vi "Destructor.vi"(8 "error in (no error)":errorcluster, 11 "Mouse in":refnum<class "Mouse.lvclass">) -> (0 "error out":errorcluster)   [LabVIEW 2021, in "InputDevice.lvlib" / "Mouse.lvclass"]
uses:
  Mouse.lvclass
  <vilib>/Utility/inputDevices.llb/closeMouse.vi
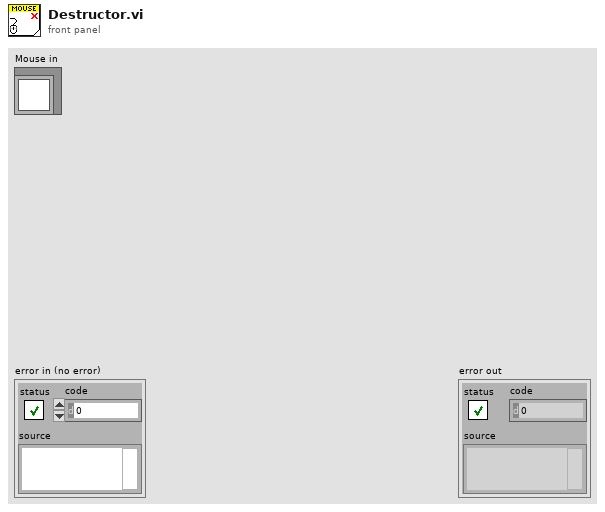
[diagram p1: front panel]
types:
  T1 = typedef "Mouse.lvclass/data.ctl" = cluster{"DeviceID":refnum<k1>, "MouseButtonInfo":refnum<user-event>, "MouseAxisInfo":refnum<user-event>, "MouseInfoEvents":refnum<event-registration>, "StopNotifier":refnum<notifier>}
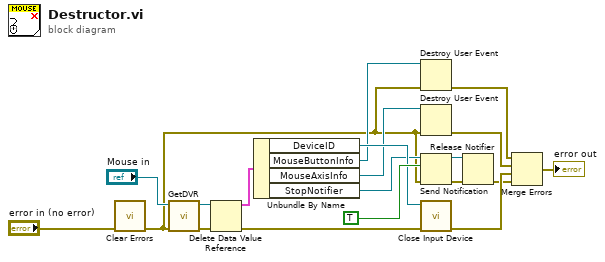
[diagram p0: block diagram]
diagram:
  n1 = call <vilib>:"Clear Errors.vi"("error in (no error)"="error in (no error)") -> ("error out"=w1:errorcluster)  [unwired: 5 in, 1 out]
  n2 = call "GetDVR.vi"("error in (no error)"=w1, "Mouse"="Mouse in") -> ("error out"=w11:errorcluster, "DVR"=w17:refnum<data-value>)  [unwired: 8 in]
  n3 = Delete Data Value Reference(data value reference=w17, error in=w11) -> (data value=w16:T1, error out=w10:errorcluster)
  n4 = Unbundle By Name(w16) -> ("DeviceID"=w15:refnum<k1>, "MouseButtonInfo"=w9:refnum<user-event>, "MouseAxisInfo"=w8:refnum<user-event>, "StopNotifier"=w7:refnum<notifier>)
  n5 = Destroy User Event(user event=w9, error in=w1) -> (error out=w6:errorcluster)
  n6 = Destroy User Event(user event=w8, error in=w1) -> (error out=w5:errorcluster)
  n7 = Send Notification(notification=TRUE, notifier=w7, error in (no error)=w1) -> (notifier out=w12:refnum<notifier>, error out=w13:errorcluster)
  n8 = call-poly <vilib>:"Close Input Device.vi"("error in (no error)"=w10, "device ID"=w15) -> ("error out"=w4:errorcluster)  [unwired: 8 in]
  n9 = Release Notifier(notifier=w12, error in (no error)=w13) -> (error out=w3:errorcluster)  [unwired: 1 in, 2 out]
  n10 = Merge Errors(w6, w5, w4, w3) -> (→"error out":errorcluster)
